vi "Aim.vi"(7 "Description":string, 8 "Command Info In":T1, 9 "Hood":dbl, 11 "Turret":dbl) -> (0 "Command Info Out":T1)   [LabVIEW 2019]
doc: "This template is useful for immediate subsystem actions that do not need deadband filtering\n\nBe sure to right-click and select New from Template and save with a new command name."
uses:
  <vilib>/Rock Robotics/WPI/Framework/Command Status Info.ctl
  <vilib>/Rock Robotics/WPI/Framework/Completion Status.ctl
  <vilib>/Rock Robotics/WPI/Framework/Completion Notifier.ctl
  Implementation/Aim Setpoints.ctl
  Implementation/Aim Operations.ctl
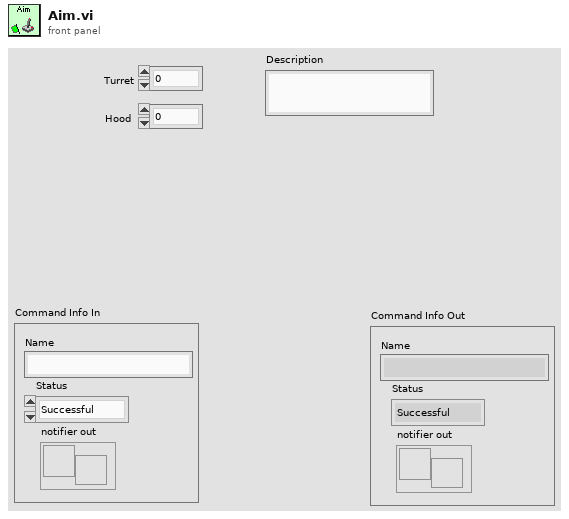
[diagram p1: front panel]
types:
  T1 = typedef "Command Status Info.ctl" = cluster{"Name":string, "Status":T2, "notifier out":T3}
  T2 = typedef "Completion Status.ctl" = enum16{"Successful", "Aborted", "Incomplete"}
  T3 = typedef "Completion Notifier.ctl" = refnum<notifier>
  T4 = typedef "Aim Setpoints.ctl" = cluster{"Operation":T5, "Turret":dbl, "Duration":dbl, "Hood":dbl}
  T5 = typedef "Aim Operations.ctl" = enum16{"Reserve", "Read Current", "Immediate", "Aim"}
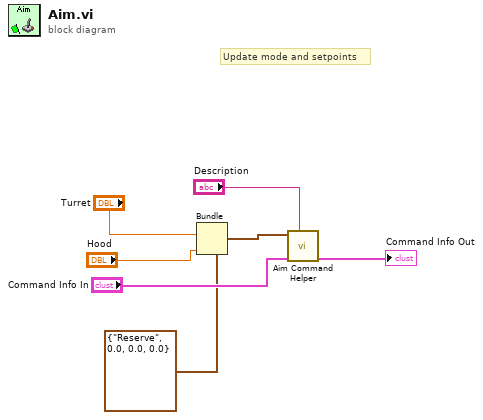
[diagram p0: block diagram]
diagram:
  # "Update mode and setpoints"
  n1 = Bundle(cluster=T4 {"Operation"=enum."Reserve", "Turret"=0.0, "Duration"=0.0, "Hood"=0.0} ("SubSystem Data"), "Turret"="Turret", "Hood"="Hood") -> (w2:T4)  [unwired: 2 in]
  n2 = call "Aim Command Helper.vi"("Description"="Description", "Command Info In"="Command Info In", "SubSystem Data"=w2) -> ("Command Info Out"=→"Command Info Out":T1)  [unwired: 6 in, 2 out]
